vi "Initialize.vi"(7 "Serial Configuration":T2={"Baud Rate"=9600, "Parity"=0, "Data Bits"=8, "Stop Bits"=10, "Flow Control"=0} {"Flow Control" items=["None", "XON/XOFF", "RTS/CTS", "XON/XOFF & RTS/CTS", "DTR/DSR", "XON/XOFF & DTR/DSR"]; "Stop Bits" items=["1.0"=10, "1.5"=15, "2.0"=20]; "Data Bits" items=["7"=7, "8"=8]; "Parity" items=["None", "Odd", "Even", "Mark", "Space"]; "Baud Rate" items=["300"=300, "600"=600, "1200"=1200, "2400"=2400, "4800"=4800, "9600"=9600, "19200"=19200]}, 8 "error in (no error)":errorcluster, 9 "Reset (True)":bool=TRUE, 10 "ID Query (True)":bool=TRUE, 11 "VISA resource name":refnum<visa-resource-name>) -> (0 "error out":errorcluster, 1 "Source Range":T1, 2 "Instrument Name":string, 3 "VISA resource name out":refnum<visa-resource-name>)   [LabVIEW 2020, in "Keithley 24XX.lvlib"]
doc: "Establishes communication with the instrument and optionally performs an instrument identification query and/or an instrument reset. It also places the instrument in a default state needed for other instrument driver operations. Therefore, call this VI before calling other instrument driver VIs for this instrument. Generally, you need to call the Initialize VI only once at the beginning of an application."
uses:
  <instrlib>/Keithley 24XX/Keithley 24XX.lvlib
panel:
  # "(c) 2006 - 2015 National Instruments.  ALL RIGHTS RESERVED."
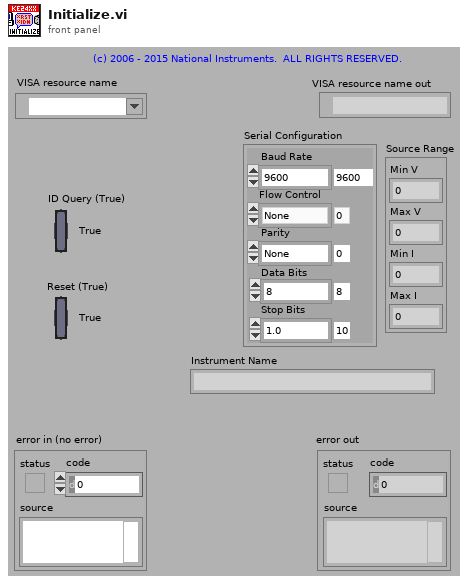
[diagram p1: front panel]
types:
  T1 = cluster{"Min V":dbl, "Max V":dbl, "Min I":dbl, "Max I":dbl}
  T2 = cluster{"Baud Rate":u32, "Parity":u16, "Data Bits":u16, "Stop Bits":u16, "Flow Control":u16}
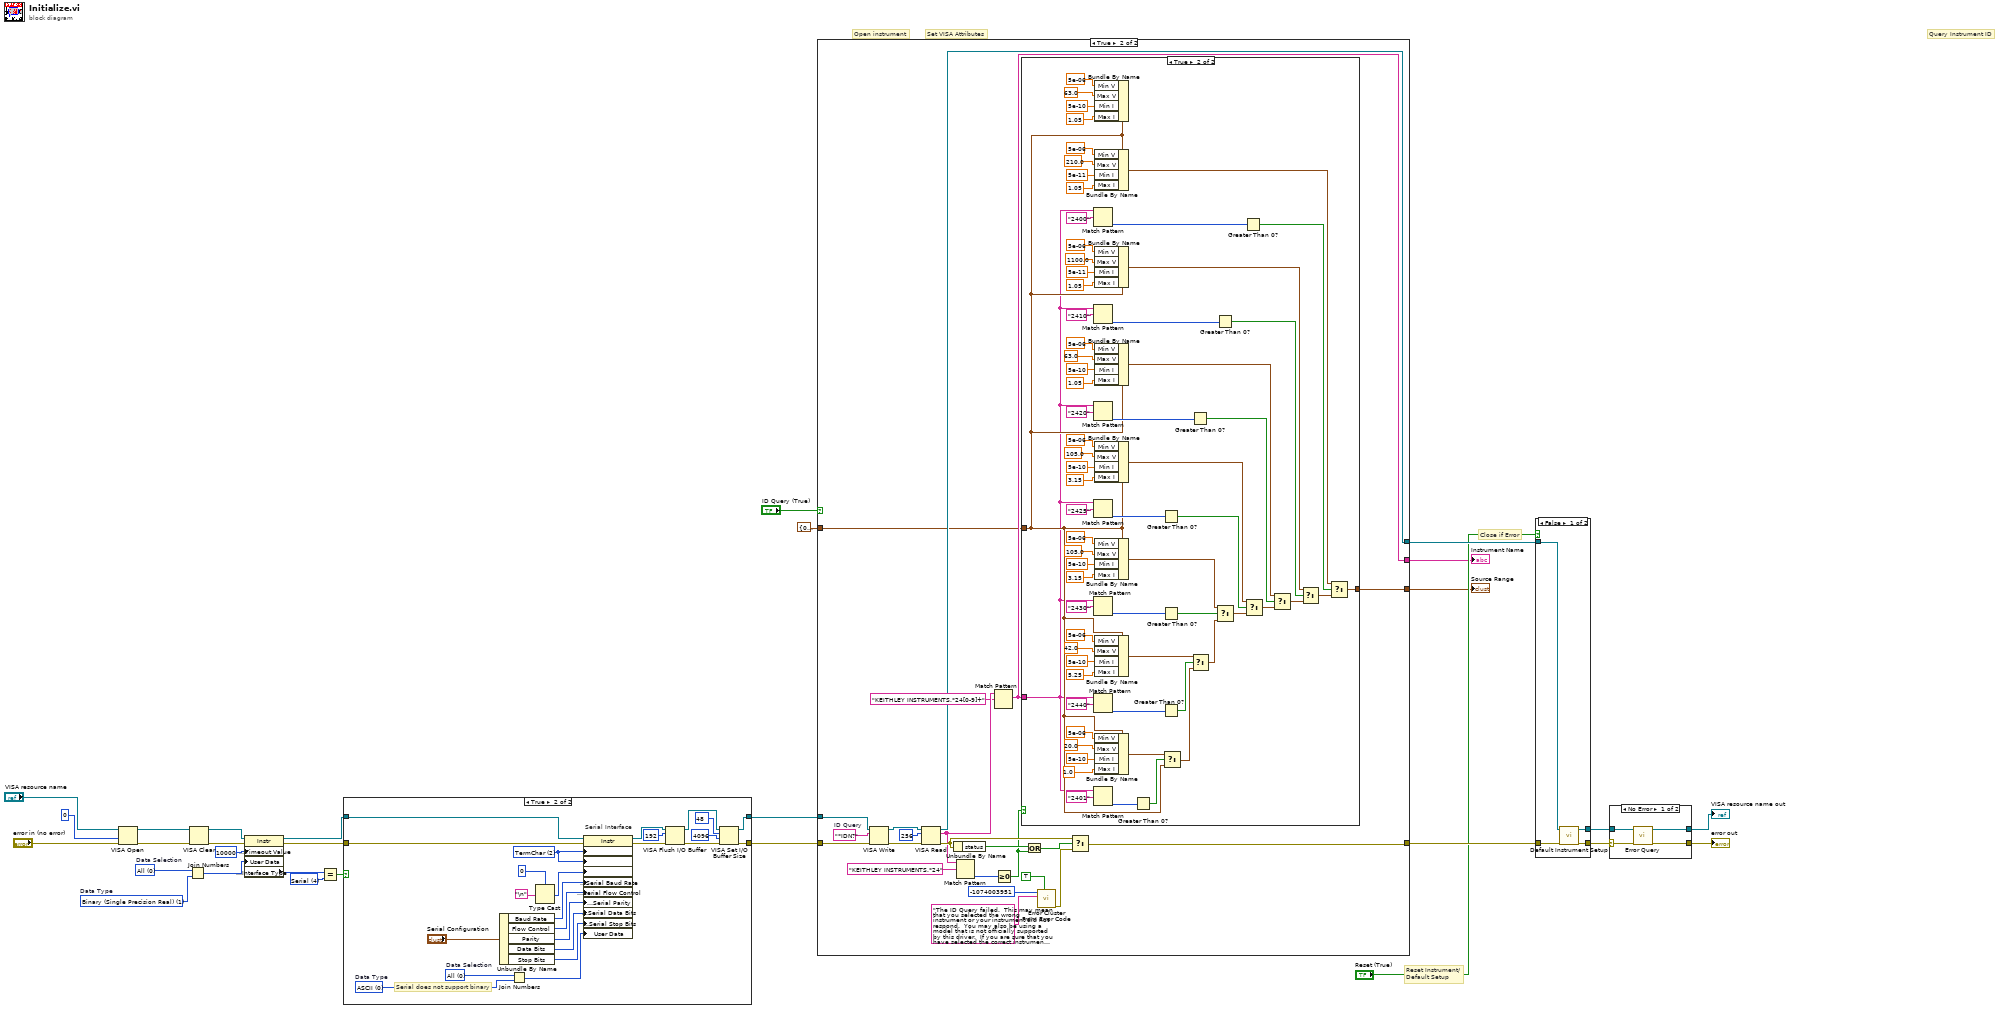
[diagram p0: block diagram]
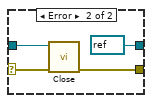
[diagram p3: hidden frame]
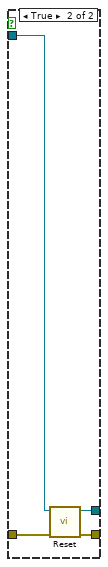
[diagram p4: hidden frame]
diagram:
  w5 = u16 1 items=["ASCII", "Binary (Single Precision Real)"]  # Data Type
  w6 = u16 0 items=["All", "Volt and Amp", "Volt", "Amp"]  # Data Selection
  w17 = u16 4 items=["GPIB"=1, "VXI"=2, "GPIB-VXI"=3, "Serial"=4, "PXI"=5, "TCPIP"=6, "USB"=7] ("Interface Information:Interface Type")
  # "Set VISA Attributes"
  # "Close if Error"
  # "Query Instrument ID"
  # "Reset Instrument/\nDefault Setup"
  # "Open instrument"
  n1 = VISA Open(access mode=u32 0, error in (no error)="error in (no error)", VISA resource name="VISA resource name") -> (VISA resource name=w15:refnum<visa-resource-name>, error out=w14:errorcluster)  [unwired: 2 in]
  n2 = Join Numbers(hi=w6, lo=w5) -> ((hi.lo)=w4:u32)
  n3 = VISA Clear(VISA resource name=w15, error in (no error)=w14) -> (VISA resource name out=w13:refnum<visa-resource-name>, error out=w12:errorcluster)
  n4 = property class="Instr"(reference=w13, error in=w12, "General Settings:Timeout Value"=u32 10000, "User Data"=w4) -> (reference out=w20:refnum<visa-resource-name>, error out=w19:errorcluster, "Interface Information:Interface Type"=w7:u16)
  n5 = Equal?(x=w7, y=w17) -> (x = y?=w18:bool)
  n6 = case shown="True" w18 {
    tunnel: [w30 w52] -> w22
    tunnel: [w31 w49] -> w21
    tunnel: w20 -> [w30 w54]
    tunnel: w19 -> [w31 w55]
    frame False {
      # "GPIB"
    }
    frame True {
      w34 = u16 0 items=["ASCII", "Binary (Single Precision Real)"]  # Data Type
      w32 = u16 0 items=["All", "Volt and Amp", "Volt", "Amp"]  # Data Selection
      w42 = u16 2 items=["None", "LastBit", "TermChar"] ("Serial Settings:Serial End Mode for Reads")
      # "Serial does not support binary"
      # "Serial Interface"
      n7 = Unbundle By Name("Serial Configuration") -> ("Baud Rate"=w40:u32, "Flow Control"=w36:u16, "Parity"=w38:u16, "Data Bits"=w39:u16, "Stop Bits"=w35:u16)
      n8 = Join Numbers(hi=w32, lo=w34) -> ((hi.lo)=w33:u32)
      n9 = Type Cast(type=u8 0, x="\n" ("Line Feed Constant")) -> (*(type *) &x=w41:u8)
      n10 = property class="Instr"(reference=w54, error in=w55, "Serial Settings:Serial End Mode for Reads"=w42, "Serial Settings:Serial End Mode for Writes"=w42, "Message Based Settings:Termination Character"=w41, "Serial Settings:Serial Baud Rate"=w40, "Serial Settings:Serial Flow Control"=w36, "Serial Settings:Serial Parity"=w38, "Serial Settings:Serial Data Bits"=w39, "Serial Settings:Serial Stop Bits"=w35, "User Data"=w33) -> (reference out=w48:refnum<visa-resource-name>, error out=w51:errorcluster)
      n11 = VISA Flush I/O Buffer(VISA resource name=w48, mask (16)=u16 192, error in (no error)=w51) -> (VISA resource name out=w53:refnum<visa-resource-name>, error out=w50:errorcluster)
      n12 = VISA Set I/O Buffer Size(VISA resource name=w53, mask (16)=u16 48, size (4096)=u32 4096 ("size (0)"), error in (no error)=w50) -> (VISA resource name out=w52:refnum<visa-resource-name>, error out=w49:errorcluster)
    }
  }
  n13 = case shown="True" "ID Query (True)" {
    tunnel: [w57 w81] -> w28
    tunnel: [w58 w78] -> w29
    tunnel: w22 -> [w58 w79]
    tunnel: w21 -> [w57 w80]
    tunnel: [_ w61] -> w3
    tunnel: [w56 w60] -> w2
    tunnel: T1 {"Min V"=0.0, "Max V"=0.0, "Min I"=0.0, "Max I"=0.0} ("input cluster") -> [w56 w59]
    frame False {
    }
    frame True {
      w73 = "*IDN?"  # ID Query
      n14 = VISA Write(VISA resource name=w79, write buffer=w73, error in (no error)=w80) -> (VISA resource name out=w77:refnum<visa-resource-name>, error out=w76:errorcluster)  [unwired: 1 out]
      n15 = VISA Read(VISA resource name=w77, byte count=u32 256, error in (no error)=w76) -> (VISA resource name out=w78:refnum<visa-resource-name>, read buffer=w64:string, error out=w67:errorcluster)  [unwired: 1 out]
      n16 = Unbundle By Name(w67) -> ("status"=w66:bool)
      n17 = Match Pattern(string=w64, regular expression="KEITHLEY INSTRUMENTS.*24") -> (offset past match=w68:i32)  [unwired: 1 in, 3 out]
      n18 = Match Pattern(string=w64, regular expression="KEITHLEY INSTRUMENTS.*24[0-9]+") -> (match substring=w61:string)  [unwired: 1 in, 3 out]
      n19 = Greater Or Equal To 0?(x=w68) -> (x >= 0?=w62:bool)
      n20 = case shown="True" w62 {
        tunnel: w61 -> [_ w83]
        tunnel: w59 -> [w82 w85]
        tunnel: [w82 w84] -> w60
        frame False {
        }
        frame True {
          n21 = Match Pattern(string=w83, regular expression="2400") -> (offset past match=w150:i32)  [unwired: 1 in, 3 out]
          n22 = Match Pattern(string=w83, regular expression="2410") -> (offset past match=w142:i32)  [unwired: 1 in, 3 out]
          n23 = Match Pattern(string=w83, regular expression="2420") -> (offset past match=w140:i32)  [unwired: 1 in, 3 out]
          n24 = Match Pattern(string=w83, regular expression="2425") -> (offset past match=w138:i32)  [unwired: 1 in, 3 out]
          n25 = Match Pattern(string=w83, regular expression="2430") -> (offset past match=w136:i32)  [unwired: 1 in, 3 out]
          n26 = Match Pattern(string=w83, regular expression="2440") -> (offset past match=w134:i32)  [unwired: 1 in, 3 out]
          n27 = Match Pattern(string=w83, regular expression="2401") -> (offset past match=w132:i32)  [unwired: 1 in, 3 out]
          n28 = Bundle By Name(cluster=w85, "Min V"=5e-06, "Max V"=63.0, "Min I"=5e-10, "Max I"=1.05 ("Max V 2")) -> ()  [unwired: 1 out]
          n29 = Bundle By Name(cluster=w85, "Min V"=5e-06, "Max V"=210.0, "Min I"=5e-11, "Max I"=1.05 ("Max V 2")) -> (w144:T1)
          n30 = Bundle By Name(cluster=w85, "Min V"=5e-06, "Max V"=1100.0, "Min I"=5e-11, "Max I"=1.05 ("Max V 2")) -> (w126:T1)
          n31 = Bundle By Name(cluster=w85, "Min V"=5e-06, "Max V"=63.0, "Min I"=5e-10, "Max I"=1.05 ("Max V 2")) -> (w115:T1)
          n32 = Bundle By Name(cluster=w85, "Min V"=5e-06, "Max V"=105.0, "Min I"=5e-10, "Max I"=3.15 ("Max V 2")) -> (w108:T1)
          n33 = Bundle By Name(cluster=w85, "Min V"=5e-06, "Max V"=105.0, "Min I"=5e-10, "Max I"=3.15 ("Max V 2")) -> (w101:T1)
          n34 = Bundle By Name(cluster=w85, "Min V"=5e-06, "Max V"=42.0, "Min I"=5e-10, "Max I"=5.25 ("Max V 2")) -> (w89:T1)
          n35 = Bundle By Name(cluster=w85, "Min V"=5e-06, "Max V"=20.0, "Min I"=5e-10, "Max I"=1.0 ("Max V 2")) -> (w87:T1)
          n36 = Greater Than 0?(x=w132) -> (x > 0?=w90:bool)
          n37 = Greater Than 0?(x=w138) -> (x > 0?=w109:bool)
          n38 = Greater Than 0?(x=w136) -> (x > 0?=w106:bool)
          n39 = Greater Than 0?(x=w134) -> (x > 0?=w91:bool)
          n40 = Select(t=w87, s=w90, f=w85) -> (s? t:f=w86:T1)
          n41 = Greater Than 0?(x=w140) -> (x > 0?=w120:bool)
          n42 = Select(t=w89, s=w91, f=w86) -> (s? t:f=w88:T1)
          n43 = Greater Than 0?(x=w142) -> (x > 0?=w131:bool)
          n44 = Select(t=w101, s=w106, f=w88) -> (s? t:f=w100:T1)
          n45 = Greater Than 0?(x=w150) -> (x > 0?=w145:bool)
          n46 = Select(t=w108, s=w109, f=w100) -> (s? t:f=w107:T1)
          n47 = Select(t=w115, s=w120, f=w107) -> (s? t:f=w114:T1)
          n48 = Select(t=w126, s=w131, f=w114) -> (s? t:f=w125:T1)
          n49 = Select(t=w144, s=w145, f=w125) -> (s? t:f=w84:T1)
        }
      }
      n50 = Or(x=w66, y=w62) -> (x .or. y?=w65:bool)
      n51 = call <vilib>:"Error Cluster From Error Code.vi"("show call chain? (False)"=TRUE, "error message (\"\")"="The ID Query failed.  This may mean that you selected the wrong instrument or your instrument did not respond.  You may also be using a model that is not officially supported by this driver.  If you are sure that you have selected the correct instrument and it is responding, try disabling the ID Query." ("Source (VI Name)"), "error code (0)"=-1074003951 ("Code")) -> ("error out"=w72:errorcluster)  [unwired: 6 in]
      n52 = Select(t=w67, s=w65, f=w72) -> (s? t:f=w81:errorcluster)
    }
  }
  "Instrument Name" <- w3
  "Source Range" <- w2
  n53 = case shown="False" "Reset (True)" {
    tunnel: w28 -> [w154 w156]
    tunnel: [w153 w159] -> w8
    tunnel: w29 -> [w155 w157]
    tunnel: [w152 w158] -> w9
    frame False {
      n54 = call <instrlib>:"Default Instrument Setup.vi"("error in (no error)"=w154, "VISA resource name"=w155) -> ("error out"=w153:errorcluster, "VISA resource name out"=w152:refnum<visa-resource-name>)  [unwired: 8 in]
    }
    frame True {
      n55 = call <instrlib>:"Reset.vi"("error in (no error)"=w156, "VISA resource name"=w157) -> ("error out"=w159:errorcluster, "VISA resource name out"=w158:refnum<visa-resource-name>)  [unwired: 8 in]
    }
  }
  n56 = case shown="No Error" w8 {
    selector: w8 -> [w161 w165]
    tunnel: w9 -> [w160 w166]
    tunnel: [w163 refnum<visa-resource-name> refnum ("VISA resource name out")] -> w11
    tunnel: [w162 w167] -> w10
    frame No Error {
      n57 = call <instrlib>:"Error Query.vi"("error in (no error)"=w161, "VISA resource name"=w160) -> ("error out"=w162:errorcluster, "VISA resource name out"=w163:refnum<visa-resource-name>)  [unwired: 6 in, 2 out]
    }
    frame Error {
      n58 = call <instrlib>:"Close.vi"("error in (no error)"=w165, "VISA resource name"=w166) -> ("error out"=w167:errorcluster)  [unwired: 9 in]
    }
  }
  "VISA resource name out" <- w11
  "error out" <- w10
